vi "Compare_Spectra_FFTs.vi"(8 "Sampling frequency":sgl=932.3896 format="%.2f", 11 "X":dbl[](array[numeric])=array[8192 elements]) -> ()   [LabVIEW 2011]
uses:
  <vilib>/Analysis/2dsp.llb/Real FFT.vi
  <vilib>/Analysis/NI_AALPro.lvlib
  <vilib>/Analysis/NI_AALBase.lvlib
panel:
  out "sum 2":dbl
  out "x*y":dbl
  out "sum":dbl
  out "u^2":dbl format="%0.4f"
  out "size(s)":i32
  out "Waveform Graph":T1(graph)
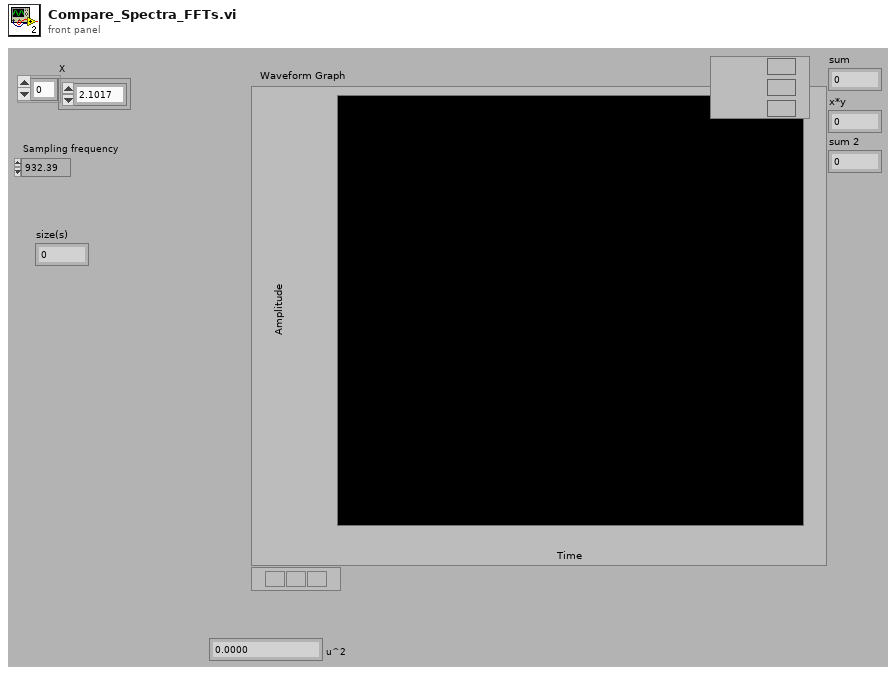
[diagram p1: front panel]
types:
  T1 = cluster{"df":dbl, "df":dbl, "Spectrum output array":dbl[]}[]
  T2 = cluster{"df":dbl, "df":dbl, "Spectrum output array":dbl[]}
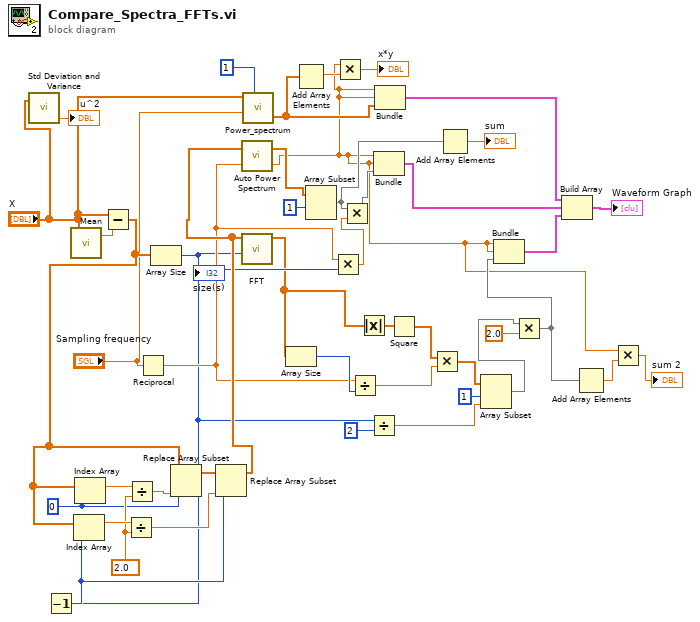
[diagram p0: block diagram]
diagram:
  w35 = 0
  w36 = 2.0
  n1 = call <vilib>:"Std Deviation and Variance.vi"("X"="X") -> ("variance"=→"u^2":dbl)  [unwired: 1 in, 2 out]
  n2 = call <vilib>:"Mean.vi"("X"="X") -> ("mean"=w42:dbl)  [unwired: 1 out]
  n3 = Subtract(x="X", y=w42) -> (x-y=w31:dbl[])
  n4 = Index Array(array=w31, index=w35) -> (element=w38:dbl)
  n5 = Divide(x=w38, y=w36) -> (x/y=w34:dbl)
  n6 = Reciprocal(x="Sampling frequency") -> (1/x=w29:sgl)
  n7 = Array Size(array=w31) -> (size(s)=w11:i32)
  "size(s)" <- w11
  n8 = Decrement(x=w11) -> (x-1=w32:i32)
  n9 = Index Array(array=w31, index=w32) -> (element=w37:dbl)
  n10 = Divide(x=w37, y=w36) -> (x/y=w33:dbl)
  n11 = Replace Array Subset(array=w31, new element=w34, index=w35) -> (w39:dbl[])
  n12 = Replace Array Subset(array=w39, new element=w33, index=w32) -> (w30:dbl[])
  n13 = call <vilib>:"Auto Power Spectrum.vi"("dt"=w29, "Signal (V)"=w30) -> ("df"=w3:dbl, "Power Spectrum (V^2 rms)"=w40:dbl[])
  n14 = call-poly <vilib>:"FFT.vi"("FFT size"=w11, "X"=w30) -> ("FFT {X}"=w8:cdb[])  [unwired: 8 in, 1 out]
  n15 = call "Power_spectrum.vi"("U"="X", "Sampling frequency"="Sampling frequency", "Block No"=1) -> ("Spectrum output array"=w20:dbl[])  [unwired: 2 in, 1 out]
  n16 = Array Size(array=w8) -> (size(s)=w45:i32)
  n17 = Add Array Elements(numeric array=w20) -> (sum=w19:dbl)
  n18 = Array Subset(array=w40, index=1) -> (w22:dbl[])  [unwired: 1 in]
  n19 = Multiply(x=w29, y=w11) -> (x*y=w13:sgl)
  n20 = Multiply(x=w3, y=w19) -> (x*y=→"x*y":dbl)
  n21 = Multiply(x=w22, y=w13) -> (x*y=w28:dbl[])
  n22 = Divide(x=w29, y=w45) -> (x/y=w44:sgl)
  n23 = Absolute Value(x=w8) -> (abs(x)=w7:dbl[])
  n24 = Divide(x=w11, y=2) -> (x/y=w9:dbl)
  n25 = Bundle("df"=w3, "df"=w3, w28) -> (w26:cluster{"df":dbl, "df":dbl, dbl[]})  [unwired: 1 in]
  n26 = Bundle("df"=w3, "df"=w3, "Spectrum output array"=w20) -> (w27:T2)  [unwired: 1 in]
  n27 = Square(x=w7) -> (x^2=w6:dbl[])
  n28 = Multiply(x=w6, y=w44) -> (x*y=w15:dbl[])
  n29 = Add Array Elements(numeric array=w22) -> (sum=→"sum":dbl)
  n30 = Array Subset(array=w15, index=1, length=w9) -> (w5:dbl[])
  n31 = Multiply(x=w5, y=sgl 2.0) -> (x*y=w4:dbl[])
  n32 = Bundle("df"=w3, "df"=w3, w4) -> (w17:cluster{"df":dbl, "df":dbl, dbl[]})  [unwired: 1 in]
  n33 = Build Array(w27, w26, w17) -> (→"Waveform Graph":T1)
  n34 = Add Array Elements(numeric array=w4) -> (sum=w2:dbl)
  n35 = Multiply(x=w3, y=w2) -> (x*y=→"sum 2":dbl)
